vi "Smart IO Switch Direction.vi"(8 "error in (no error)":errorcluster, 10 "isInput":bool, 11 "deviceIndex":i32) -> (0 "error out":errorcluster)   [LabVIEW 2026, in "MrcLib.lvlib"]
doc: "Quickly flip the direction of a digital device channel. This can be useful if bit-banging slower communication protocols."
uses:
  MrcLib.lvlib
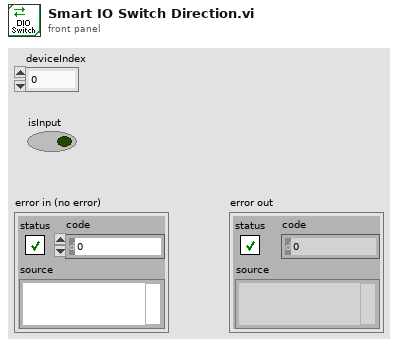
[diagram p1: front panel]
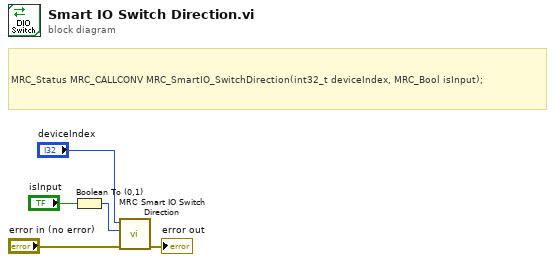
[diagram p0: block diagram]
diagram:
  # "MRC_Status MRC_CALLCONV MRC_SmartIO_SwitchDirection(int32_t deviceIndex, MRC_Bool isInput);"
  n1 = Boolean To (0,1)(Boolean="isInput") -> (0, 1=w2:i16)
  n2 = call "MRC Smart IO Switch Direction.vi"("error in (no error)"="error in (no error)", "isInput"=w2, "deviceIndex"="deviceIndex") -> ("error out"=→"error out":errorcluster)  [unwired: 8 in]
